vi "usrp set time now.vi"(7 "mboard":u64, 8 "error in (no error)":errorcluster, 9 "frac_secs":dbl, 10 "full_secs":i64, 11 "h":u64) -> (0 "error out":errorcluster, 3 "function return":u32(ring))   [LabVIEW 2023, in "uhd.lvlib"]
doc: "UHD_API uhd_error uhd_usrp_set_time_now(\n uhd_usrp_handle h, int64_t full_secs, double frac_secs, size_t mboard);"
uses:
  <userlib>/uhd/uhd.lvlib
  <userlib>/uhd/uhd.dll
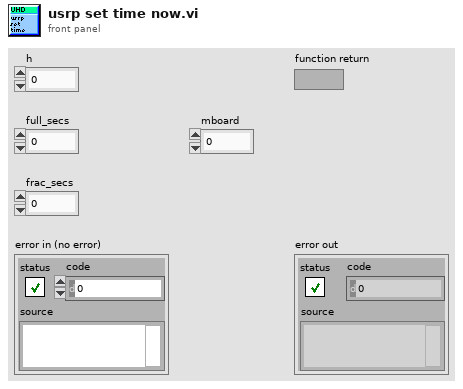
[diagram p1: front panel]
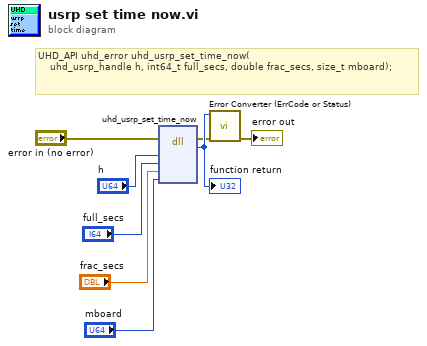
[diagram p0: block diagram]
diagram:
  # "UHD_API uhd_error uhd_usrp_set_time_now(\n    uhd_usrp_handle h, int64_t full_secs, double frac_secs, size_t mboard);"
  n1 = dll-call lib="C:/Program Files/National Instruments/LabVIEW 2023/user.lib/uhd/uhd.*" fn="uhd_usrp_set_time_now"(error in="error in (no error)", "h"="h", "full_secs"="full_secs", "frac_secs"="frac_secs", "mboard"="mboard") -> (error out=w2:errorcluster, w8:u32)  [unwired: 6 in, 1 out]
  "function return" <- w8
  n2 = call <userlib>:"Error Converter (ErrCode or Status).vi"("error in (no error)"=w2, "error code"=w8) -> ("error out"=→"error out":errorcluster)  [unwired: 9 in]
